vi "Intake Controller.vi"(8 "error in":errorcluster) -> ()   [LabVIEW 2016, in "Intake.lvlib"]
uses:
  Intake.lvlib
  Fuel/Fuel State.ctl
  <vilib>/Rock Robotics/WPI/Solenoid/WPI_SolenoidDevRef.ctl
  <vilib>/Rock Robotics/WPI/Solenoid/WPI_SolenoidChannel.ctl
  Typedef/Intake Msg.ctl
  Typedef/Intake Command.ctl
  <vilib>/Rock Robotics/WPI/RobotDrive/WPI_RobotDriveDevRef.ctl
  <vilib>/Rock Robotics/WPI/MotorControl/WPI_MotorControlDeviceRef.ctl
  <vilib>/Rock Robotics/WPI/MotorControl/WPI_MotorControlType.ctl
  <vilib>/Rock Robotics/SystemInterfaces/DIO/FPGA_DIOPWMChannel.ctl
  <vilib>/Rock Robotics/WPI/PWM/WPI_PWMDeadband.ctl
  <vilib>/Rock Robotics/WPI/AnalogChannel/WPI_AnalogChannelDevRef.ctl
  <vilib>/Rock Robotics/SystemInterfaces/AI/FPGA_AIChannel.ctl
  <vilib>/Rock Robotics/WPI/Framework/Completion Status.ctl
  <vilib>/Rock Robotics/WPI/Utilities/WPI_GetSetVariantRefNum.vi
  Constants/Private/Private Global.vi
  <vilib>/Rock Robotics/WPI/Solenoid/WPI_SolenoidSetEnum.vi
  <vilib>/addons/control/pid/pid.llb/PID Output Rate Limiter (DBL).vi
  Constants/Constants.lvlib
  <vilib>/addons/control/pid/NI_PID_pid.lvlib
panel:
  in  "Enable Test Mode":bool
  in  "Is Gear Released?":bool
  in  "Has Gear?":bool
  in  "Gear Puncher":bool
  in  "Gear Release Value":bool
  in  "Gear Wait Time":i32(slide) scale=-1.0..1.0
  in  "Fuel Arm Value":bool
  in  "Gear Flip Speed":dbl(slide) scale=-1.0..1.0
  in  "Front Roller Speed":dbl(slide) scale=-1.0..1.0
  in  "Roller Rate Limit":dbl(slide) scale=-1.0..200.0
  in  "Fuel Roller Speed":dbl(slide) scale=-1.0..1.0
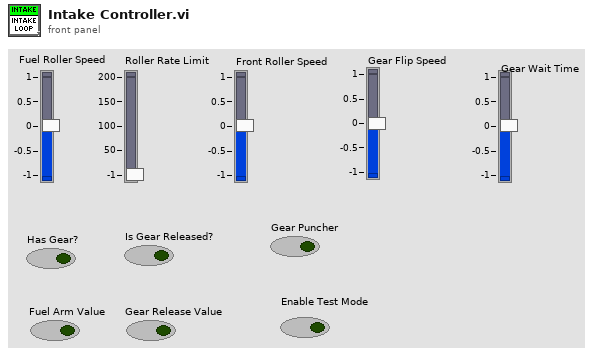
[diagram p1: front panel]
types:
  T1 = typedef "Intake.lvlib/Intake Command.ctl" = enum16{"Gear On", "Gear Off", "Gear Reverse", "Gear Retract", "Gear Deploy", "Gear Push Up", "All Off", "All Off Closed", "Fuel Deploy", "Fuel Retract", "Fuel Agitate", "Fuel Reverse"}
  T2 = typedef "Intake.lvlib/Fuel State.ctl" = cluster{"Deployed?":bool, "Fuel Roller Speed":dbl, "Front Roller Speed":dbl}
  T3 = typedef "WPI_SolenoidDevRef.ctl" = cluster{"DevStatus":errorcluster, "Pneumatics Control Module":u8, "Forward Solenoid Channel":T4, "Reverse Solenoid Channel":T4}
  T4 = typedef "WPI_SolenoidChannel.ctl" = enum8{"Solenoid 0", "Solenoid 1", "Solenoid 2", "Solenoid 3", "Solenoid 4", "Solenoid 5", "Solenoid 6", "Solenoid 7", "Invalid"}
  T5 = typedef "WPI_RobotDriveDevRef.ctl" = cluster{"DevStatus":errorcluster, "Motors[]":T6[], "Square Inputs":bool, "Max Output":dbl}
  T6 = typedef "WPI_MotorControlDeviceRef.ctl" = cluster{"DeviceStatus":errorcluster, "Type":T7, "PWM":cluster{"PWM Channel":T8, "DeadBand":T9}, "CAN":cluster{"Device Number":u8, "SetOutput VI Ref":variant, "GetOutput VI Ref":variant, "Enable VI Ref":variant, "Disable VI Ref":variant, "Data":variant}, "Invert":bool}
  T7 = typedef "WPI_MotorControlType.ctl" = enum16{"PWM", "CAN"}
  T8 = typedef "FPGA_DIOPWMChannel.ctl" = enum8{"PWM 0", "PWM 1", "PWM 2", "PWM 3", "PWM 4", "PWM 5", "PWM 6", "PWM 7", "PWM 8", "PWM 9", "PWM MXP 0", "PWM MXP 1", "PWM MXP 2", "PWM MXP 3", "PWM MXP 4", "PWM MXP 5", "PWM MXP 6", "PWM MXP 7", "PWM MXP 8", "PWM MXP 9", "Invalid"}
  T9 = typedef "WPI_PWMDeadband.ctl" = cluster{"Name":string, "maxPositivePwm":i32, "minPositivePwm":i32, "centerPwm":i32, "maxNegativePwm":i32, "minNegativePwm":i32, "angularRange":u16}
  T10 = typedef "WPI_AnalogChannelDevRef.ctl" = cluster{"DevStatus":errorcluster, "Analog Channel":T11}
  T11 = typedef "FPGA_AIChannel.ctl" = enum8{"AI 0", "AI 1", "AI 2", "AI 3", "AI MXP 0", "AI MXP 1", "AI MXP 2", "AI MXP 3", "Invalid"}
  T12 = cluster{"Fuel State":T2, "Fuel Arm":T3, "queue":refnum<queue>, "Fuel Roller":T5, "Front Roller":T6, "Gear Release":T3, "Gear Flip":T6, "Gear Release Value":bool, "Fuel Roller Speed":dbl, "Front Roller Speed":dbl, "Gear Flip Speed":dbl, "Fuel Arm Value":bool, "Gear Wait Time":i32, "Has Gear?":bool, "Is Gear Released?":bool, "Gear Sensor":T10, "Roller Rate Limit":dbl, "Gear Puncher":T3, "Gear Puncher Value":bool}
  T13 = typedef "Completion Status.ctl" = enum16{"Successful", "Aborted", "Incomplete"}
  T14 = typedef "Intake.lvlib/Intake Msg.ctl" = cluster{"Cmd":T1, "Variant":variant}
  T15 = typedef "Constants.lvlib/Constants.ctl" = cluster{"Port Layout":cluster{"RightMotorInverted":bool, "LeftMotorInverted":bool, "Left Motors":T8, "Right Motors":T8, "Auton List":string[], "XBOX Port":T16, "Encoder L A":T17, "Encoder L B":T17, "Encoder R A":T17, "Encoder R B":T17, "L Encoder Inverse":bool, "R Encoder Inverse":bool, "Drive Distance per Count":dbl, "Gyro Bus":T18, "Fuel Roller 1":T8, "Front Roller":T8, "Gear Flipper":T8, "Climber 1":T8, "Fuel Roller Invert":bool, "Front Roller Invert":bool, "Gear Flipper Invert":bool, "Climber Invert":bool, "PCM":u8, "Fuel Roller 2":T8, "Gear Sensor":T11, "Gear Release Fwd":T4, "Gear Release Rvrs":T4, "Fuel Arm Fwd":T4, "Fuel Arm Rvrs":T4, "Shifter Fwrd":T4, "Shifter Rvrs":T4, "Climber 2":T8, "PDP":u8, "Shooter Front Channel":u8, "Shooter Rear Channel":u8, "Shooter Feed Channel":u8, "Camera Servo":T8, "Gear Servo":T8, "Gear Puncher Fwrd":T4, "Gear Puncher Rvrs":T4, "Shooter Inverse":bool, "Ring Light Switch":T17}, "Drive Constants":cluster{"Wheelbase In.":dbl, "Max Velocity (In/sec)":dbl, "Max Accel (In/sec^2)":dbl, "Max Jerk (In/sec^3)":dbl, "Path dt":dbl, "Path Sample Count":i32, "Deadband":dbl}, "Arm System":cluster{"Front Roller Gear Speed":dbl, "Front Roller Fuel Speed":dbl, "Gear Flipper Speed":dbl, "Fuel Roller Speed":dbl, "Gear Release Wait (ms)":i32, "Gear Sensor Threshold":dbl, "Flappy Open Angle":i32, "Flappy Close Angle":i32, "Ramp Rate (EGU/min)":dbl}, "Shooter":cluster{"Shooter Wheels":cluster{"P":dbl, "I":dbl, "D":dbl, "F":dbl, "IZone":dbl}, "Feeder":cluster{"P":dbl, "I":dbl, "D":dbl, "F":dbl, "IZone":dbl}, "Front Shooter RPM":dbl, "Rear Shooter RPM":dbl, "Agitator Speed":dbl, "Feeder Speed":dbl, "Shooter CPR":u32, "Feeder CPR":u32}, "Vision":cluster{"High Goal Height (in.)":dbl, "Low Goal Height (in.)":dbl, "Camera Height High (in.)":dbl, "Camera Height Low (in.)":dbl, "Servo Pitch Gear (deg)":dbl, "Camera Yaw (deg)":dbl, "Servo Gear":i32, "Servo Boiler":i32, "Servo Pitch Boiler (deg)":dbl}}
  T16 = typedef "WPI_JoystickDeviceEnum.ctl" = enum16{"USB 0", "USB 1", "USB 2", "USB 3", "USB 4", "USB 5"}
  T17 = typedef "FPGA_DIOChannel.ctl" = enum8{"DIO 0", "DIO 1", "DIO 2", "DIO 3", "DIO 4", "DIO 5", "DIO 6", "DIO 7", "DIO 8", "DIO 9", "DIO MXP 0", "DIO MXP 1", "DIO MXP 2", "DIO MXP 3", "DIO MXP 4", "DIO MXP 5", "DIO MXP 6", "DIO MXP 7", "DIO MXP 8", "DIO MXP 9", "DIO MXP 10", "DIO MXP 11", "DIO MXP 12", "DIO MXP 13", "DIO MXP 14", "DIO MXP 15", "SPI Port CS1", "SPI Port CS2", "SPI Port CS3", "SPI Port MISO", "SPI Port MOSI", "Invalid"}
  T18 = typedef "spi_bus.ctl" = enum16{"SPI On-Board, CS0", "SPI On-Board, CS1", "SPI On-Board, CS2", "SPI On-Board, CS3", "SPI MXP", "Invalid"}
  T19 = typedef "WPI_SolenoidValue.ctl" = enum16{"Off", "On", "Forward", "Reverse"}
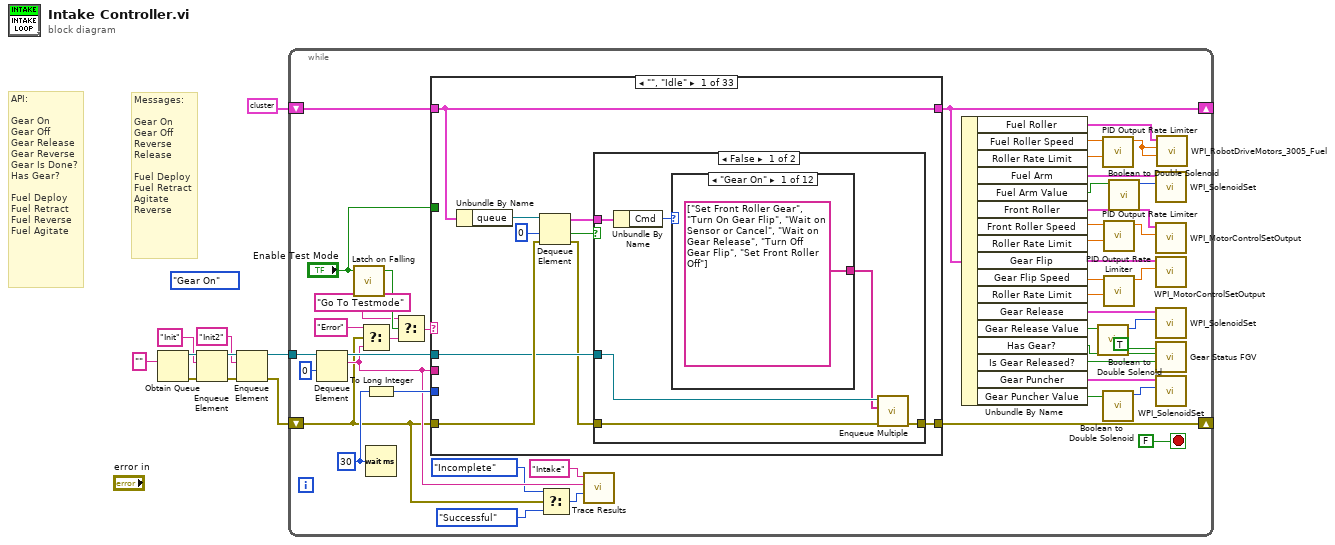
[diagram p0: block diagram]
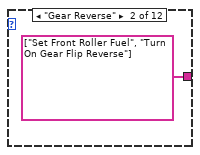
[diagram p2: hidden frame]
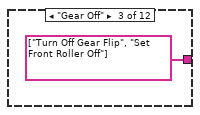
[diagram p3: hidden frame]
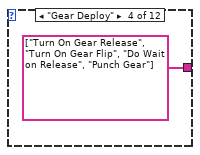
[diagram p4: hidden frame]
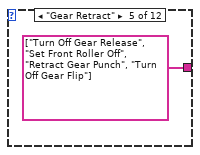
[diagram p5: hidden frame]
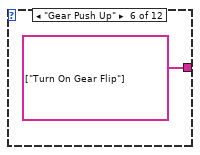
[diagram p6: hidden frame]
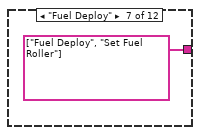
[diagram p7: hidden frame]
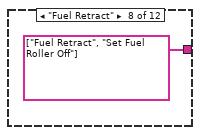
[diagram p8: hidden frame]
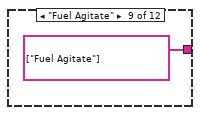
[diagram p9: hidden frame]
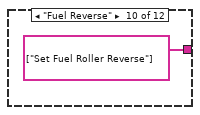
[diagram p10: hidden frame]
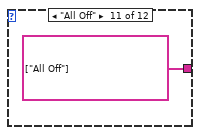
[diagram p11: hidden frame]
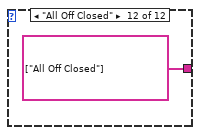
[diagram p12: hidden frame]
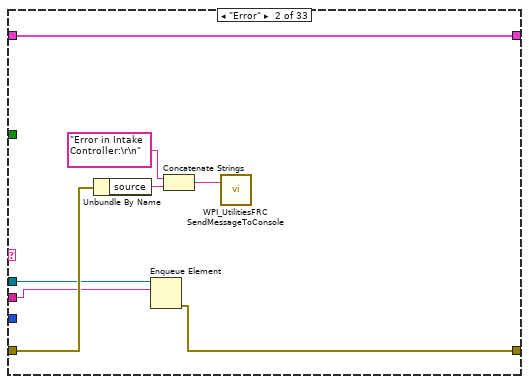
[diagram p14: hidden frame]
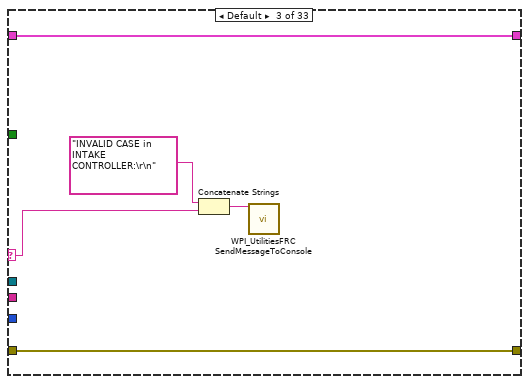
[diagram p15: hidden frame]
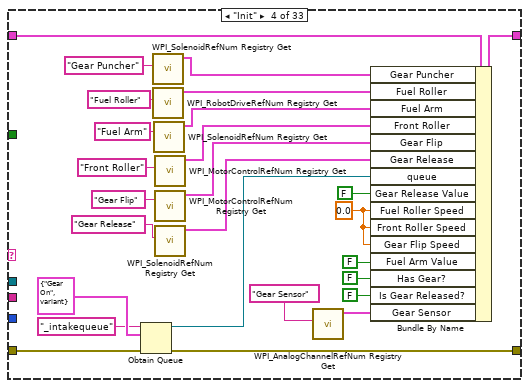
[diagram p16: hidden frame]
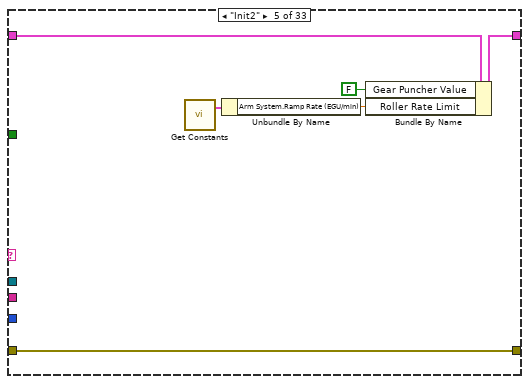
[diagram p17: hidden frame]
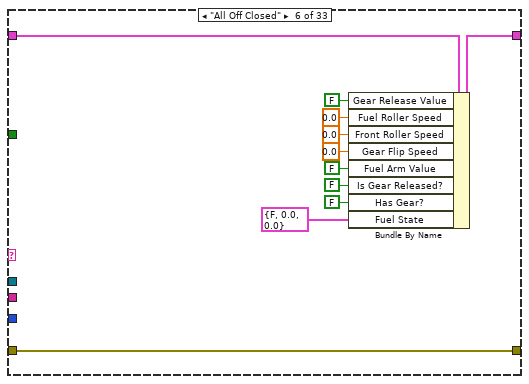
[diagram p18: hidden frame]
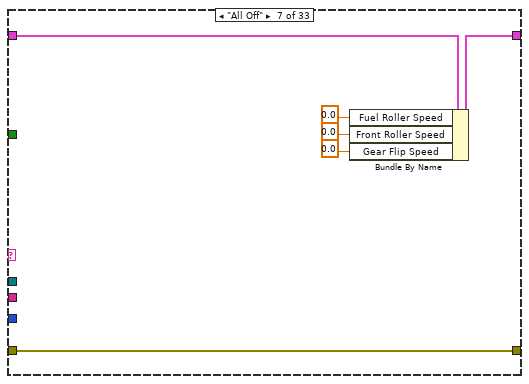
[diagram p19: hidden frame]
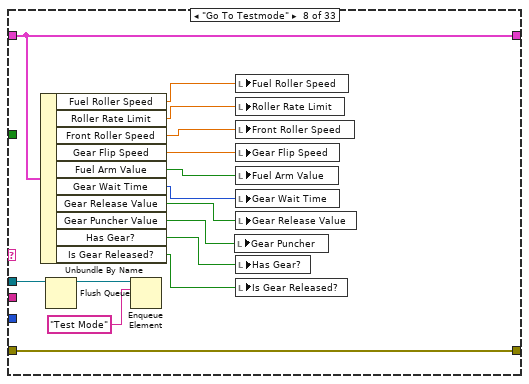
[diagram p20: hidden frame]
diagram:
  (unwired) Intake_Command."Gear On" ("Cmd")
  # "API:\n\nGear On\nGear Off\nGear Release\nGear Reverse\nGear Is Done?\nHas Gear?\n\nFuel Deploy\nFuel Retract\nFuel Reverse\nFuel Agitate"
  # "Messages:\n\nGear On\nGear Off\nReverse\nRelease\n\nFuel Deploy\nFuel Retract\nAgitate\nReverse"
  n1 = Obtain Queue(element data type="") -> (queue out=w8:refnum<queue>, error out=w9:errorcluster)  [unwired: 4 in, 1 out]
  n2 = Enqueue Element(queue=w8, element="Init", error in (no error)=w9) -> (queue out=w3:refnum<queue>, error out=w5:errorcluster)  [unwired: 1 in, 1 out]
  n3 = Enqueue Element(queue=w3, element="Init2", error in (no error)=w5) -> (queue out=w2:refnum<queue>, error out=w4:errorcluster)  [unwired: 1 in, 1 out]
  n4 = while {
    shift-right: [w53] -> _
    shift-left: T12 {"Fuel State"={"Deployed?"=FALSE, "Fuel Roller Speed"=0.0, "Front Roller Speed"=0.0}, "Fuel Arm"={"DevStatus"={"status"=FALSE, "code"=0, "source"=""}, "Pneumatics Control Module"=0, "Forward Solenoid Channel"=enum."Solenoid 0", "Reverse Solenoid Channel"=enum."Solenoid 0"}, "queue"=refnum, "Fuel Roller"={"DevStatus"={"status"=FALSE, "code"=0, "source"=""}, "Motors[]"=[], "Square Inputs"=FALSE, "Max Output"=1.0}, "Front Roller"={"DeviceStatus"={"status"=FALSE, "code"=0, "source"=""}, "Type"=enum."PWM", "PWM"={"PWM Channel"=enum."Invalid", "DeadBand"={"Name"="", "maxPositivePwm"=0, "minPositivePwm"=0, "centerPwm"=0, "maxNegativePwm"=0, "minNegativePwm"=0, "angularRange"=0}}, "CAN"={"Device Number"=0, "SetOutput VI Ref"=variant(refnum<vi> refnum), "GetOutput VI Ref"=variant(refnum<vi> refnum), "Enable VI Ref"=variant(refnum<vi> refnum), "Disable VI Ref"=variant(refnum<vi> refnum), "Data"=variant}, "Invert"=FALSE}, "Gear Release"={"DevStatus"={"status"=FALSE, "code"=0, "source"=""}, "Pneumatics Control Module"=0, "Forward Solenoid Channel"=enum."Solenoid 0", "Reverse Solenoid Channel"=enum."Solenoid 0"}, "Gear Flip"={"DeviceStatus"={"status"=FALSE, "code"=0, "source"=""}, "Type"=enum."PWM", "PWM"={"PWM Channel"=enum."Invalid", "DeadBand"={"Name"="", "maxPositivePwm"=0, "minPositivePwm"=0, "centerPwm"=0, "maxNegativePwm"=0, "minNegativePwm"=0, "angularRange"=0}}, "CAN"={"Device Number"=0, "SetOutput VI Ref"=variant(refnum<vi> refnum), "GetOutput VI Ref"=variant(refnum<vi> refnum), "Enable VI Ref"=variant(refnum<vi> refnum), "Disable VI Ref"=variant(refnum<vi> refnum), "Data"=variant}, "Invert"=FALSE}, "Gear Release Value"=FALSE, "Fuel Roller Speed"=0.0, "Front Roller Speed"=0.0, "Gear Flip Speed"=0.0, "Fuel Arm Value"=FALSE, "Gear Wait Time"=0, "Has Gear?"=FALSE, "Is Gear Released?"=FALSE, "Gear Sensor"={"DevStatus"={"status"=FALSE, "code"=0, "source"=""}, "Analog Channel"=enum."Invalid"}, "Roller Rate Limit"=0.0, "Gear Puncher"={"DevStatus"={"status"=FALSE, "code"=0, "source"=""}, "Pneumatics Control Module"=0, "Forward Solenoid Channel"=enum."Invalid", "Reverse Solenoid Channel"=enum."Invalid"}, "Gear Puncher Value"=FALSE} ("cluster") -> [w55]
    shift-right: [w54] -> _
    shift-left: w4 -> [w38]
    tunnel: w2 -> [w50]
    stop <- FALSE stop-if-true
    w42 = u32 30 ("milliseconds to wait")
    n5 = Dequeue Element(queue=w50, timeout in ms (-1)=0) -> (queue out=w48:refnum<queue>, element=w40:string)  [unwired: 1 in, 2 out]
    n6 = call "Latch on Falling.vi"("Boolean in"="Enable Test Mode") -> ("Boolean out"=w14:bool)  [unwired: 4 in]
    n7 = Select(t="Error", s=w38, f=w40) -> (s? t:f=w15:string)
    n8 = To Long Integer(number=w42) -> (32bit integer=w41:i32)
    n9 = Wait (ms)(milliseconds to wait=w42) -> ()  [unwired: 1 out]
    n10 = Select(t="Go To Testmode", s=w14, f=w15) -> (s? t:f=w13:string)
    n11 = case shown="\"\", \"Idle\"" w13 {
      selector: w13 -> [_ _ w92 _ _ _ _ _ _ _ _ _ _ _ _ _ _ _ _ _ _ _ _ _ _ _ _ _ _ _ _ _ _]
      tunnel: w55 -> [w64 w91 w96 w120 w128 w139 w145 w159 w175 w180 w184 w190 w197 w202 w207 w213 w217 w227 w239 w244 w250 w259 w270 w277 w281 w283 w288 w292 w298 w303 w307 w311 w315]
      tunnel: [w64 w91 w96 w119 w126 w137 w143 w159 w173 w180 w185 w191 w195 w200 w205 w211 w215 w228 w239 w242 w248 w255 w268 w275 w279 w283 w286 w290 w296 w301 w305 w309 w313] -> w53
      tunnel: [w56 w84 w95 w118 w127 w138 w144 w160 w174 w179 w186 w192 w196 w201 w206 w212 w216 w230 w238 w243 w249 w258 w271 w276 w280 w282 w287 w291 w297 w302 w306 w310 w314] -> w54
      tunnel: w38 -> [w61 w90 w95 w117 w127 w138 w144 w160 w174 w179 w186 w192 w196 w201 w206 w212 w216 w230 w238 w243 w249 w258 w271 w276 w280 w282 w287 w291 w297 w302 w306 w310 w314]
      tunnel: w48 -> [w58 w86 _ _ _ _ _ w147 w162 _ _ _ _ _ _ _ _ w229 _ _ _ w257 w269 _ _ _ _ _ _ _ _ _ _]
      tunnel: w40 -> [_ w85 _ _ _ _ _ _ _ _ _ _ _ _ _ _ _ _ _ _ _ _ _ _ _ _ _ _ _ _ _ _ _]
      tunnel: w41 -> [_ _ _ _ _ _ _ _ _ _ _ _ _ _ _ _ _ _ _ _ _ w252 w266 _ _ _ _ _ _ _ _ _ _]
      tunnel: "Enable Test Mode" -> [_ _ _ _ _ _ _ _ w161 _ _ _ _ _ _ _ _ _ _ _ _ _ _ _ _ _ _ _ _ _ _ _ _]
      frame "", "Idle" {
        n12 = Unbundle By Name(w64) -> ("queue"=w63:refnum<queue>)
        n13 = Dequeue Element(queue=w63, timeout in ms (-1)=0, error in (no error)=w61) -> (element=w60:T14, timed out?=w59:bool, error out=w57:errorcluster)  [unwired: 1 out]
        n14 = case shown="False" w59 {
          tunnel: w60 -> [w70 _]
          tunnel: w58 -> [w66 _]
          tunnel: w57 -> [w67 w83]
          tunnel: [w68 w83] -> w56
          frame False {
            n15 = Unbundle By Name(w70) -> ("Cmd"=w69:T1)
            n16 = case shown="\"Gear On\"" w69 {
              tunnel: [string[] ["Set Front Roller Gear", "Turn On Gear Flip", "Wait on Sensor or Cancel", "Wait on Gear Release", "Turn Off Gear Flip", "Set Front Roller Off"] string[] ["Set Front Roller Fuel", "Turn On Gear Flip Reverse"] string[] ["Turn Off Gear Flip", "Set Front Roller Off"] string[] ["Turn On Gear Release", "Turn On Gear Flip", "Do Wait on Release", "Punch Gear"] string[] ["Turn Off Gear Release", "Set Front Roller Off", "Retract Gear Punch", "Turn Off Gear Flip"] string[] ["Turn On Gear Flip"] string[] ["Fuel Deploy", "Set Fuel Roller"] string[] ["Fuel Retract", "Set Fuel Roller Off"] string[] ["Fuel Agitate"] string[] ["Set Fuel Roller Reverse"] string[] ["All Off"] string[] ["All Off Closed"]] -> w65
              frame "Gear On" {
              }
              frame "Gear Reverse" {
              }
              frame "Gear Off" {
              }
              frame "Gear Deploy" {
              }
              frame "Gear Retract" {
              }
              frame "Gear Push Up" {
              }
              frame "Fuel Deploy" {
              }
              frame "Fuel Retract" {
              }
              frame "Fuel Agitate" {
              }
              frame "Fuel Reverse" {
              }
              frame "All Off" {
              }
              frame "All Off Closed" {
              }
            }
            n17 = call "Enqueue Multiple.vi"("error in (no error)"=w67, "Array"=w65, "Queue in"=w66) -> ("error out"=w68:errorcluster)  [unwired: 8 in]
          }
          frame True {
            # "No new command"
          }
        }
      }
      frame "Error" {
        n18 = Unbundle By Name(w90) -> ("source"=w89:string)
        n19 = Enqueue Element(queue=w86, element=w85) -> (error out=w84:errorcluster)  [unwired: 2 in, 2 out]
        n20 = Concatenate Strings("Error in Intake Controller:\r\n" ("string"), w89) -> (w88:string)
        n21 = call <vilib>:"WPI_UtilitiesFRC SendMessageToConsole.vi"("Message"=w88) -> ()  [unwired: 14 in, 1 out]
      }
      frame Default {
        n22 = Concatenate Strings("INVALID CASE in INTAKE CONTROLLER:\r\n" ("string"), w92) -> (w93:string)
        n23 = call <vilib>:"WPI_UtilitiesFRC SendMessageToConsole.vi"("Message"=w93) -> ()  [unwired: 14 in, 1 out]
      }
      frame "Init" {
        w103 = 0.0 ("Fuel Roller Speed")
        n24 = Obtain Queue(name (unnamed)="_intakequeue", element data type=T14 {"Cmd"=enum."Gear On", "Variant"=variant}, error in (no error)=w117) -> (queue out=w106:refnum<queue>, error out=w118:errorcluster)  [unwired: 2 in, 1 out]
        n25 = call <vilib>:"WPI_SolenoidRefNum Registry Get.vi"("refnum name"="Gear Puncher") -> ("SolenoidDevRef"=w97:T3)  [unwired: 9 in, 1 out]
        n26 = call <vilib>:"WPI_RobotDriveRefNum Registry Get.vi"("refnum name"="Fuel Roller") -> ("RobotDriveDevRef"=w116:T5)  [unwired: 9 in, 1 out]
        n27 = call <vilib>:"WPI_SolenoidRefNum Registry Get.vi"("refnum name"="Fuel Arm") -> ("SolenoidDevRef"=w113:T3)  [unwired: 9 in, 1 out]
        n28 = call <vilib>:"WPI_MotorControlRefNum Registry Get.vi"("refnum name"="Front Roller") -> ("MotorControlDevRef"=w111:T6)  [unwired: 9 in, 1 out]
        n29 = call <vilib>:"WPI_MotorControlRefNum Registry Get.vi"("refnum name"="Gear Flip") -> ("MotorControlDevRef"=w109:T6)  [unwired: 9 in, 1 out]
        n30 = call <vilib>:"WPI_SolenoidRefNum Registry Get.vi"("refnum name"="Gear Release") -> ("SolenoidDevRef"=w107:T3)  [unwired: 9 in, 1 out]
        n31 = call <vilib>:"WPI_AnalogChannelRefNum Registry Get.vi"("refnum name"="Gear Sensor") -> ("AIDeviceRef"=w99:T10)  [unwired: 9 in, 1 out]
        n32 = Bundle By Name(cluster=w120, "Gear Puncher"=w97, "Fuel Roller"=w116, "Fuel Arm"=w113, "Front Roller"=w111, "Gear Flip"=w109, "Gear Release"=w107, "queue"=w106, "Gear Release Value"=FALSE ("Gear Release"), "Fuel Roller Speed"=w103, "Front Roller Speed"=w103, "Gear Flip Speed"=w103, "Fuel Arm Value"=FALSE ("Fuel Arm"), "Has Gear?"=FALSE, "Is Gear Released?"=FALSE, "Gear Sensor"=w99) -> (w119:T12)
      }
      frame "Init2" {
        n33 = call "Get Constants.vi"() -> ("Constants"=w125:T15)  [unwired: 3 in]
        n34 = Unbundle By Name(w125) -> ("Arm System.Ramp Rate (EGU/min)"=w124:dbl)
        n35 = Bundle By Name(cluster=w128, "Gear Puncher Value"=FALSE, "Roller Rate Limit"=w124) -> (w126:T12)
      }
      frame "All Off Closed" {
        n36 = Bundle By Name(cluster=w139, "Gear Release Value"=FALSE, "Fuel Roller Speed"=0.0, "Front Roller Speed"=0.0, "Gear Flip Speed"=0.0, "Fuel Arm Value"=FALSE, "Is Gear Released?"=FALSE, "Has Gear?"=FALSE, "Fuel State"=T2 {"Deployed?"=FALSE, "Fuel Roller Speed"=0.0, "Front Roller Speed"=0.0}) -> (w137:T12)
      }
      frame "All Off" {
        n37 = Bundle By Name(cluster=w145, "Fuel Roller Speed"=0.0, "Front Roller Speed"=0.0, "Gear Flip Speed"=0.0) -> (w143:T12)
      }
      frame "Go To Testmode" {
        n38 = Unbundle By Name(w159) -> ("Fuel Roller Speed"=w158:dbl, "Roller Rate Limit"=w157:dbl, "Front Roller Speed"=w156:dbl, "Gear Flip Speed"=w155:dbl, "Fuel Arm Value"=w154:bool, "Gear Wait Time"=w153:i32, "Gear Release Value"=w151:bool, "Gear Puncher Value"=w152:bool, "Has Gear?"=w150:bool, "Is Gear Released?"=w149:bool)
        n39 = Flush Queue(queue=w147) -> (queue out=w146:refnum<queue>)  [unwired: 1 in, 2 out]
        n40 = Enqueue Element(queue=w146, element="Test Mode") -> ()  [unwired: 2 in, 3 out]
        n41 = local write "Gear Puncher"(w152) -> ()
        n42 = local write "Fuel Roller Speed"(w158) -> ()
        n43 = local write "Roller Rate Limit"(w157) -> ()
        n44 = local write "Front Roller Speed"(w156) -> ()
        n45 = local write "Gear Flip Speed"(w155) -> ()
        n46 = local write "Fuel Arm Value"(w154) -> ()
        n47 = local write "Gear Wait Time"(w153) -> ()
        n48 = local write "Gear Release Value"(w151) -> ()
        n49 = local write "Has Gear?"(w150) -> ()
        n50 = local write "Is Gear Released?"(w149) -> ()
      }
      frame "Test Mode" {
        n51 = case shown="True" w161 {
          tunnel: w162 -> [_ w177]
          frame False {
          }
          frame True {
            n52 = Flush Queue(queue=w177) -> (queue out=w176:refnum<queue>)  [unwired: 1 in, 2 out]
            n53 = Enqueue Element(queue=w176, element="Test Mode") -> ()  [unwired: 2 in, 3 out]
          }
        }
        n54 = Bundle By Name(cluster=w175, "Fuel Arm Value"="Fuel Arm Value", "Front Roller Speed"="Front Roller Speed", "Fuel Roller Speed"="Fuel Roller Speed", "Roller Rate Limit"="Roller Rate Limit", "Gear Flip Speed"="Gear Flip Speed", "Gear Wait Time"="Gear Wait Time", "Gear Release Value"="Gear Release Value", "Gear Puncher Value"="Gear Puncher", "Has Gear?"="Has Gear?", "Is Gear Released?"="Is Gear Released?") -> (w173:T12)
      }
      frame "/**** Gear Intake Actions ***/" {
        # "Do not use this case"
      }
      frame "Store Fuel State" {
        n55 = Unbundle By Name(w184) -> ("Fuel Arm Value"=w183:bool, "Fuel Roller Speed"=w182:dbl, "Front Roller Speed"=w181:dbl)
        n56 = Bundle By Name(cluster=w184, "Fuel State.Deployed?"=w183, "Fuel State.Fuel Roller Speed"=w182, "Fuel State.Front Roller Speed"=w181) -> (w185:T12)
      }
      frame "Restore Fuel State" {
        n57 = Unbundle By Name(w190) -> ("Fuel State.Deployed?"=w189:bool, "Fuel State.Fuel Roller Speed"=w188:dbl, "Fuel State.Front Roller Speed"=w187:dbl)
        n58 = Bundle By Name(cluster=w190, "Fuel Arm Value"=w189, "Fuel Roller Speed"=w188, "Front Roller Speed"=w187) -> (w191:T12)
      }
      frame "Turn Off Fuel" {
        n59 = Bundle By Name(cluster=w197, "Fuel Arm Value"=FALSE, "Fuel Roller Speed"=0.0) -> (w195:T12)
      }
      frame "Set Front Roller Gear" {
        n60 = call "Get Constants.vi"() -> ("Constants"=w199:T15)  [unwired: 3 in]
        n61 = Unbundle By Name(w199) -> ("Arm System.Front Roller Gear Speed"=w198:dbl)
        n62 = Bundle By Name(cluster=w202, "Front Roller Speed"=w198) -> (w200:T12)
      }
      frame "Turn On Gear Flip" {
        n63 = call "Get Constants.vi"() -> ("Constants"=w204:T15)  [unwired: 3 in]
        n64 = Unbundle By Name(w204) -> ("Arm System.Gear Flipper Speed"=w203:dbl)
        n65 = Bundle By Name(cluster=w207, "Gear Flip Speed"=w203) -> (w205:T12)
      }
      frame "Turn On Gear Flip Reverse" {
        n66 = call "Get Constants.vi"() -> ("Constants"=w210:T15)  [unwired: 3 in]
        n67 = Unbundle By Name(w210) -> ("Arm System.Gear Flipper Speed"=w209:dbl)
        n68 = Negate(x=w209) -> (-x=w208:dbl)
        n69 = Bundle By Name(cluster=w213, "Gear Flip Speed"=w208) -> (w211:T12)
      }
      frame "Turn Off Gear Flip" {
        n70 = Bundle By Name(cluster=w217, "Gear Flip Speed"=0.0) -> (w215:T12)
      }
      frame "Wait on Sensor or Cancel" {
        n71 = call "Get Constants.vi"() -> ("Constants"=w222:T15)  [unwired: 3 in]
        n72 = Unbundle By Name(w227) -> ("queue"=w226:refnum<queue>, "Gear Sensor"=w220:T10)
        n73 = Unbundle By Name(w222) -> ("Arm System.Gear Sensor Threshold"=w221:dbl)
        n74 = call <vilib>:"WPI_AnalogChannelGetAverageVoltage.vi"("AIDeviceRef"=w220) -> ("Voltage"=w219:dbl)  [unwired: 8 in, 2 out]
        n75 = Get Queue Status(queue=w226) -> (# elements in queue=w218:i32)  [unwired: 2 in, 7 out]
        n76 = Greater Than 0?(x=w218) -> (x > 0?=w225:bool)
        n77 = Greater?(x=w219, y=w221) -> (0:w223:bool)
        n78 = Or(x=w225, y=w223) -> (x .or. y?=w224:bool)
        n79 = case shown="False" w224 {
          tunnel: w229 -> [w233 _]
          tunnel: w227 -> [w231 w237]
          tunnel: [w231 w236] -> w228
          tunnel: w223 -> [_ w235]
          frame False {
            n80 = Enqueue Element At Opposite End(queue=w233, element="Wait on Sensor or Cancel") -> ()  [unwired: 2 in, 3 out]
          }
          frame True {
            n81 = Not(x=w235) -> (.not. x?=w234:bool)
            n82 = Bundle By Name(cluster=w237, "Has Gear?"=w235, "Is Gear Released?"=w234) -> (w236:T12)
          }
        }
      }
      frame "/*** Gear Release Actions ***/" {
      }
      frame "Turn On Gear Release" {
        n83 = Bundle By Name(cluster=w244, "Gear Release Value"=TRUE, "Is Gear Released?"=FALSE) -> (w242:T12)
      }
      frame "Turn Off Gear Release" {
        n84 = Bundle By Name(cluster=w250, "Gear Release Value"=FALSE, "Has Gear?"=FALSE, "Is Gear Released?"=TRUE) -> (w248:T12)
      }
      frame "Wait on Gear Release" {
        n85 = call "Get Constants.vi"() -> ("Constants"=w256:T15)  [unwired: 3 in]
        n86 = Unbundle By Name(w256) -> ("Arm System.Gear Release Wait (ms)"=w254:i32)
        n87 = Subtract(x=w254, y=w252) -> (x-y=w253:i32)
        n88 = Bundle By Name(cluster=w259, "Gear Wait Time"=w253) -> (w255:T12)
        n89 = Enqueue Element At Opposite End(queue=w257, element="Do Wait on Release") -> ()  [unwired: 2 in, 3 out]
      }
      frame "Do Wait on Release" {
        # "up to +30ms of jitter from set time random, not critical here"
        n90 = Unbundle By Name(w270) -> ("queue"=w261:refnum<queue>, "Gear Wait Time"=w267:i32)
        n91 = Subtract(x=w267, y=w266) -> (x-y=w265:i32)
        n92 = Get Queue Status(queue=w261) -> (# elements in queue=w260:i32)  [unwired: 2 in, 7 out]
        n93 = Less Or Equal To 0?(x=w265) -> (x <= 0?=w264:bool)
        n94 = Greater Than 0?(x=w260) -> (x > 0?=w262:bool)
        n95 = Or(x=w262, y=w264) -> (x .or. y?=w263:bool)
        n96 = case shown="False" w263 {
          tunnel: w269 -> [w273 _]
          frame False {
            n97 = Enqueue Element At Opposite End(queue=w273, element="Do Wait on Release") -> ()  [unwired: 2 in, 3 out]
          }
          frame True {
          }
        }
        n98 = Bundle By Name(cluster=w270, "Gear Wait Time"=w265) -> (w268:T12)
      }
      frame "Retract Gear Punch" {
        n99 = Bundle By Name(cluster=w277, "Gear Puncher Value"=FALSE) -> (w275:T12)
      }
      frame "Punch Gear" {
        n100 = Bundle By Name(cluster=w281, "Gear Puncher Value"=TRUE) -> (w279:T12)
      }
      frame "/*** Fuel Actions **/" {
      }
      frame "Set Front Roller Fuel" {
        n101 = call "Get Constants.vi"() -> ("Constants"=w285:T15)  [unwired: 3 in]
        n102 = Unbundle By Name(w285) -> ("Arm System.Front Roller Fuel Speed"=w284:dbl)
        n103 = Bundle By Name(cluster=w288, "Front Roller Speed"=w284) -> (w286:T12)
      }
      frame "Set Front Roller Off" {
        n104 = Bundle By Name(cluster=w292, "Front Roller Speed"=0.0 ("Fuel Roller Speed")) -> (w290:T12)
      }
      frame "Set Fuel Roller Reverse" {
        n105 = call "Get Constants.vi"() -> ("Constants"=w295:T15)  [unwired: 3 in]
        n106 = Unbundle By Name(w295) -> ("Arm System.Fuel Roller Speed"=w294:dbl)
        n107 = Negate(x=w294) -> (-x=w293:dbl)
        n108 = Bundle By Name(cluster=w298, "Fuel Roller Speed"=w293) -> (w296:T12)
      }
      frame "Set Fuel Roller" {
        n109 = call "Get Constants.vi"() -> ("Constants"=w300:T15)  [unwired: 3 in]
        n110 = Unbundle By Name(w300) -> ("Arm System.Fuel Roller Speed"=w299:dbl)
        n111 = Bundle By Name(cluster=w303, "Fuel Roller Speed"=w299) -> (w301:T12)
      }
      frame "Set Fuel Roller Off" {
        n112 = Bundle By Name(cluster=w307, "Fuel Roller Speed"=0.0) -> (w305:T12)
      }
      frame "Fuel Deploy" {
        n113 = Bundle By Name(cluster=w311, "Fuel Arm Value"=TRUE) -> (w309:T12)
      }
      frame "Fuel Retract" {
        n114 = Bundle By Name(cluster=w315, "Fuel Arm Value"=FALSE) -> (w313:T12)
      }
    }
    n115 = Select(t=Completion_Status."Incomplete" ("Status of previous command"), s=w38, f=Completion_Status."Successful" ("Status of previous command")) -> (s? t:f=w35:T13)
    n116 = call <vilib>:"Trace Results.vi"("Status of previous command"=w35, "Description"=w40, "Subsystem"="Intake") -> ()  [unwired: 9 in]
    n117 = Unbundle By Name(w53) -> ("Fuel Roller"=w28:T5, "Fuel Roller Speed"=w26:dbl, "Roller Rate Limit"=w25:dbl, "Fuel Arm"=w52:T3, "Fuel Arm Value"=w43:bool, "Front Roller"=w46:T6, "Front Roller Speed"=w23:dbl, "Roller Rate Limit"=w22:dbl, "Gear Flip"=w45:T6, "Gear Flip Speed"=w20:dbl, "Roller Rate Limit"=w19:dbl, "Gear Release"=w44:T3, "Gear Release Value"=w31:bool, "Has Gear?"=w34:bool, "Is Gear Released?"=w33:bool, "Gear Puncher"=w18:T3, "Gear Puncher Value"=w17:bool)
    n118 = call "Boolean to Double Solenoid.vi"("Dir?"=w31) -> ("Value"=w30:T19)  [unwired: 10 in]
    n119 = call-poly <vilib>:"PID Output Rate Limiter.vi"("output rate (EGU/min)"=w25, "input (controller output)"=w26) -> ("output"=w27:dbl)  [unwired: 6 in, 1 out]
    n120 = call "Boolean to Double Solenoid.vi"("Dir?"=w17) -> ("Value"=w16:T19)  [unwired: 10 in]
    n121 = call-poly <vilib>:"PID Output Rate Limiter.vi"("output rate (EGU/min)"=w22, "input (controller output)"=w23) -> ("output"=w24:dbl)  [unwired: 6 in, 1 out]
    n122 = call-poly <vilib>:"PID Output Rate Limiter.vi"("output rate (EGU/min)"=w19, "input (controller output)"=w20) -> ("output"=w21:dbl)  [unwired: 6 in, 1 out]
    n123 = call "Boolean to Double Solenoid.vi"("Dir?"=w43) -> ("Value"=w29:T19)  [unwired: 10 in]
    n124 = call-poly <vilib>:"WPI_SolenoidSet.vi"("Value"=w29, "SolenoidDevRef"=w52) -> ()  [unwired: 8 in, 2 out]
    n125 = call <vilib>:"WPI_MotorControlSetOutput.vi"("Output"=w24, "MotorControlDevRef"=w46) -> ()  [unwired: 7 in, 3 out]
    n126 = call <vilib>:"WPI_MotorControlSetOutput.vi"("Output"=w21, "MotorControlDevRef"=w45) -> ()  [unwired: 7 in, 3 out]
    n127 = call-poly <vilib>:"WPI_SolenoidSet.vi"("Value"=w30, "SolenoidDevRef"=w44) -> ()  [unwired: 8 in, 2 out]
    n128 = call "Gear Status FGV.vi"("Is Gear Released?"=w33, "Has Gear?"=w34, "Set? (F)"=TRUE) -> ()  [unwired: 6 in, 3 out]
    n129 = call-poly <vilib>:"WPI_SolenoidSet.vi"("Value"=w16, "SolenoidDevRef"=w18) -> ()  [unwired: 8 in, 2 out]
    n130 = call "WPI_RobotDriveMotors_3005_Fuel.vi"("RightSpeed"=w27, "LeftSpeed"=w27, "RobotDriveDevRef"=w28) -> ()  [unwired: 6 in, 3 out]
  }
